vi "Z_valve_state.vi"(0 "Z_Source":T1(ring), 1 "ZM_State":u32, 5 "Z_SetState":T2(ring)=enum."on", 7 "Alarm_L1":bool, 9 "Alarm_L2":bool, 12 "TsStop":u32=1000, 13 "t_check":u32=10000) -> (4 "Z_Source_Out":T1(ring), 6 "Z_State":T2(ring), 8 "t":u32)   [LabVIEW 2019, in "Valves.lvlib"]
uses:
  Valves.lvlib
  Trigers/RS.vi
  Timer Delay/Timer.vi
  Userlib.lvlib
panel:
  in  "t2_tmp":u32[][](array[numeric])=[[0, 0], [0, 0], [0, 0], [0, 0], [0, 0], [0, 0], [0, 0], [0, 0], [0, 0], [0, 0], [0, 0], [0, 0], [0, 0]]
  in  "C2_tmp":cluster{"C":bool, "NC":u32}[][](array[cluster])
  in  "t_tmp":u32[][](array[numeric])=[[0, 0], [0, 0], [0, 0], [0, 0], [0, 0], [0, 0], [0, 0], [0, 0], [0, 0], [0, 0], [0, 0], [0, 0], [0, 0]]
  in  "C_tmp":cluster{"C":bool, "NC":u32}[][](array[cluster])
  # "Temporally arrays"
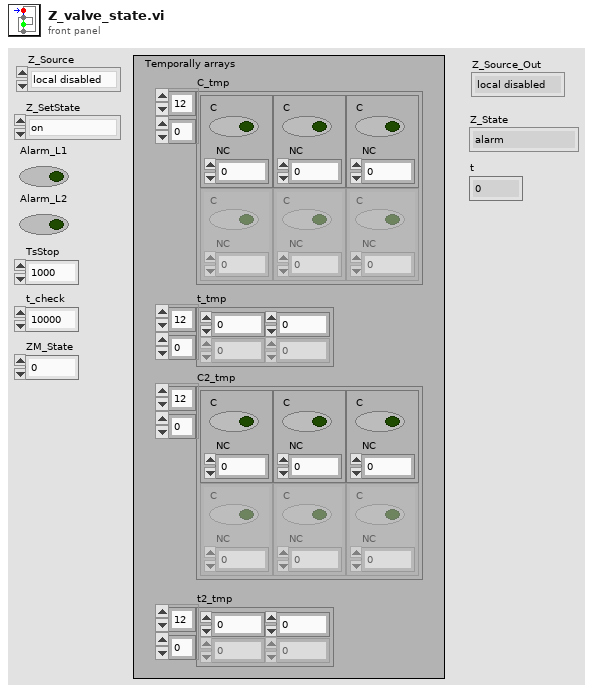
[diagram p1: front panel]
types:
  T1 = enum8{"local disabled", "local hand", "hand", "auto", "dist"}
  T2 = enum8{"alarm", "disabled", "not ready", "stop ready", "reserv", "switched off", "switched on", "check", "on min", "decrease speed", "on", "increase speed", "on max"}
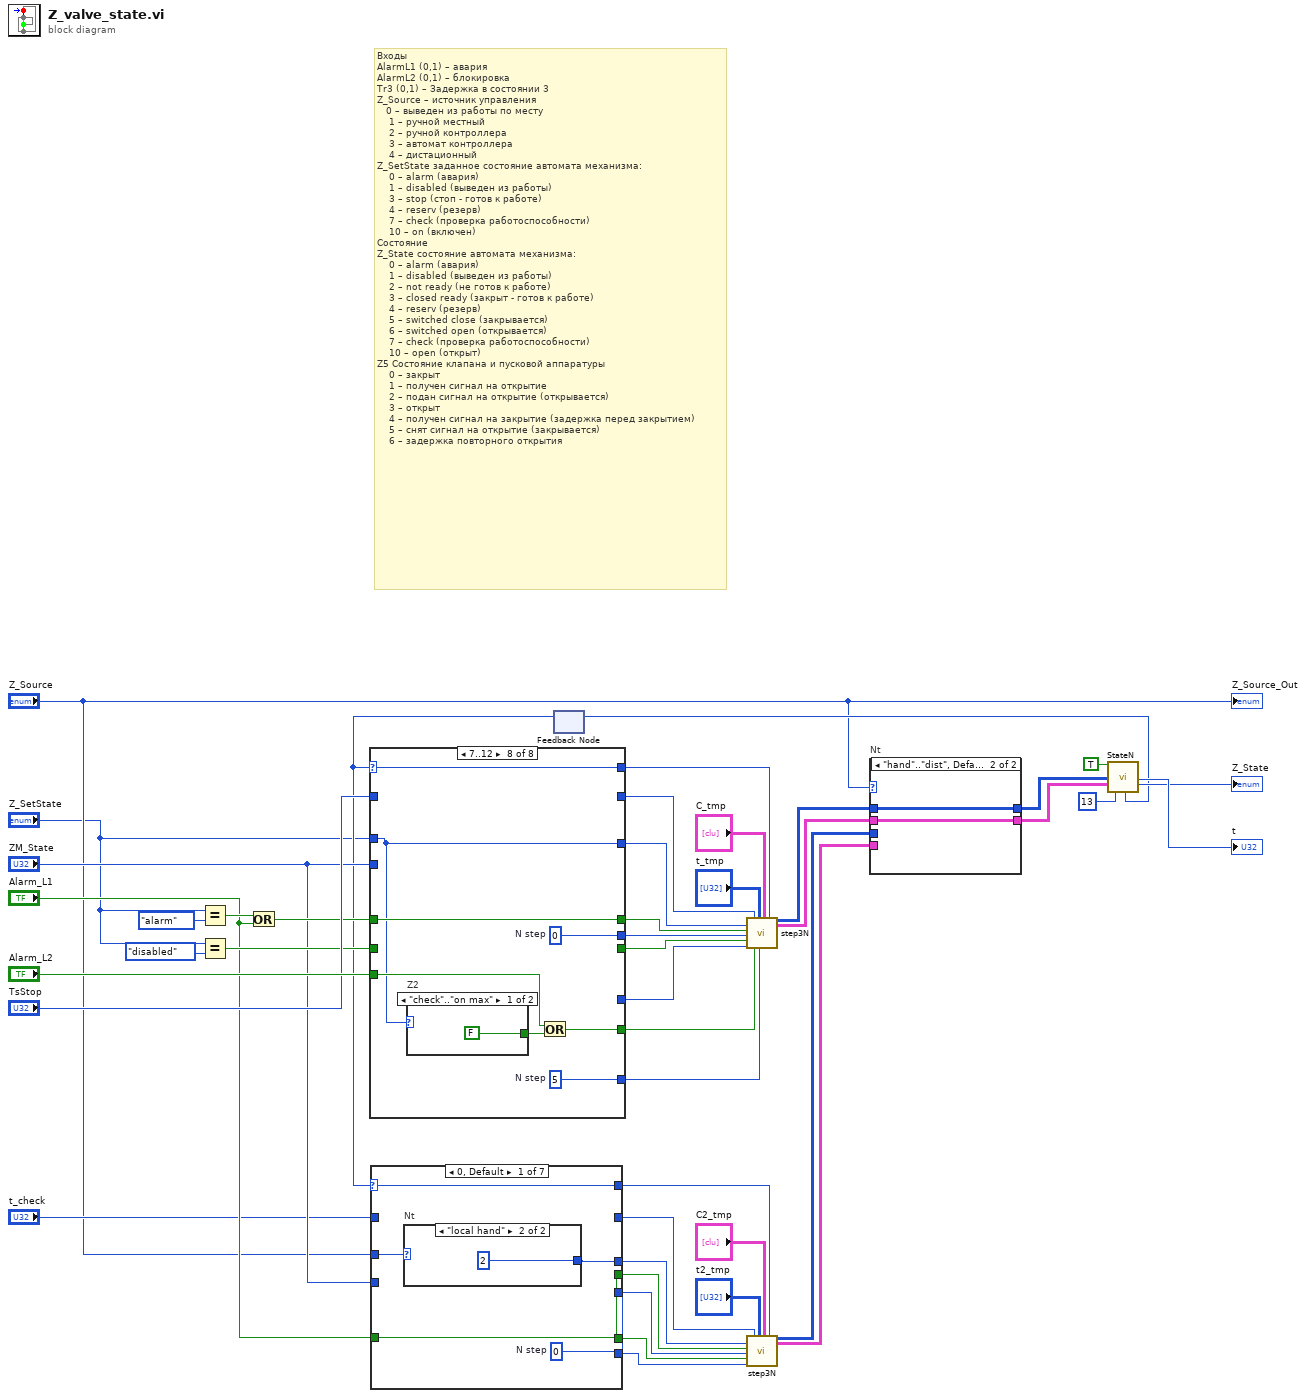
[diagram p0: block diagram]
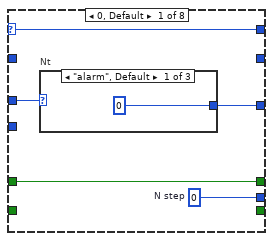
[diagram p2: hidden frame]
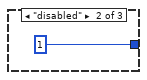
[diagram p3: hidden frame]
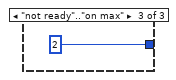
[diagram p4: hidden frame]
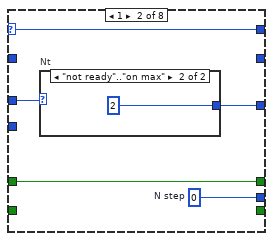
[diagram p5: hidden frame]
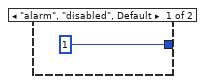
[diagram p6: hidden frame]
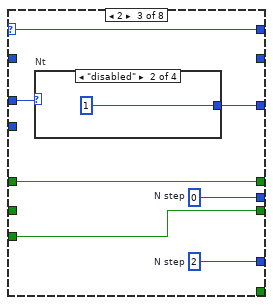
[diagram p7: hidden frame]
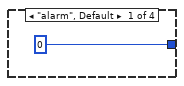
[diagram p8: hidden frame]
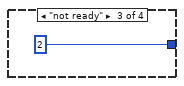
[diagram p9: hidden frame]
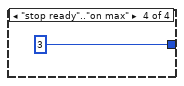
[diagram p10: hidden frame]
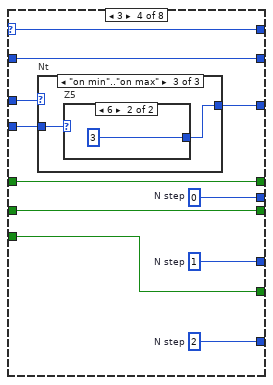
[diagram p11: hidden frame]
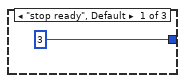
[diagram p12: hidden frame]
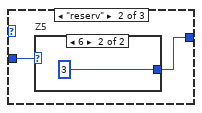
[diagram p13: hidden frame]
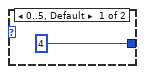
[diagram p14: hidden frame]
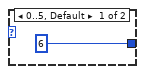
[diagram p15: hidden frame]
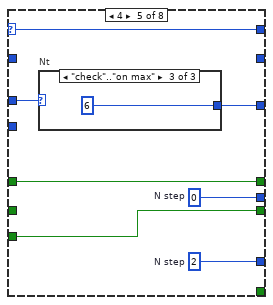
[diagram p16: hidden frame]
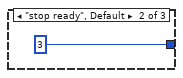
[diagram p18: hidden frame]
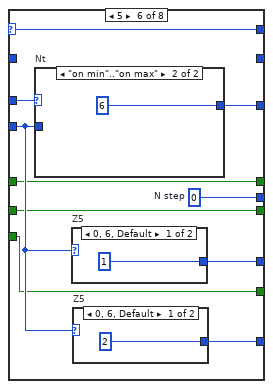
[diagram p19: hidden frame]
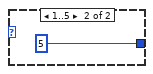
[diagram p20: hidden frame]
diagram:
  # "Входы\nAlarmL1 (0,1) – авария\nAlarmL2 (0,1) – блокировка\nTr3 (0,1) – Задержка в состоянии 3\nZ_Source – источник управления\n   0 – выведен из работы по месту\n    1 – ручной местный\n    2 – ручной контроллера\n    3 – автомат контроллера\n    4 – дистационный\nZ_SetState заданное состояние автомата механизма:\n    0 – alarm (авария)\n    1 – disabled (выведен из работы)\n    3 – stop (стоп - готов к работе)\n    4 – reserv (резерв)\n    7 – check (проверка работоспособности)\n    10 – on (включен)\nСостояние\nZ_State состояние автомата механизма:\n    0 – alarm (авария)\n    1 – disabled (выведен из работы)\n    2 – not ready (не готов к работе)\n    3 – closed ready (закрыт - готов к работе)\n    4 – reserv (резерв)\n    5 – switched close (закрывается)\n    6 – switched open (открывается)\n    7 – check (проверка работоспособности)\n    10 – open (открыт)\nZ5 Состояние клапана и пусковой аппаратуры\n    0 – закрыт\n    1 – получен сигнал на открытие\n    2 – подан сигнал на открытие (открывается)\n    3 – открыт\n    4 – получен сигнал на закрытие (задержка перед закрытием)\n    5 – снят сигнал на открытие (закрывается)\n    6 – задержка повторного открытия"
  n1 = Equal?(x="Z_SetState", y=T2."alarm") -> (x = y?=w44:bool)
  n2 = Equal?(x="Z_SetState", y=T2."disabled") -> (x = y?=w33:bool)
  n3 = Or(x=w44, y="Alarm_L1") -> (x .or. y?=w32:bool)
  n4 = feedback #1() -> (w7:u32)  [unwired: 1 in]
  n5 = case shown="7..12" w7 {
    selector: w7 -> [w47 w55 w62 w80 w97 w102 w126 w135]
    tunnel: w32 -> [w48 w56 w63 w73 w92 w103 w121 w139]
    tunnel: "Alarm_L2" -> [_ _ w65 w77 w94 w107 w127 w141]
    tunnel: "ZM_State" -> [_ _ _ w81 _ w110 w129 _]
    tunnel: "TsStop" -> [_ _ _ w79 _ _ _ _]
    tunnel: w33 -> [_ _ _ w75 _ w105 _ _]
    tunnel: [w47 w55 w62 w80 w97 w102 w126 w135] -> w18
    tunnel: [w48 w56 w63 w73 w92 w103 w121 w139] -> w25
    tunnel: [w49 w57 w64 w74 w93 w104 w122 w138] -> w24
    tunnel: [_ _ _ w77 _ w107 w124 w137] -> w20
    tunnel: [_ _ _ w78 _ w108 w123 w136] -> w19
    tunnel: [w46 w54 w61 w72 w96 w109 w125 w134] -> w23
    tunnel: [_ _ w66 w76 w95 w106 _ _] -> w22
    tunnel: [_ _ w65 w75 w94 w105 _ _] -> w21
    tunnel: [_ _ _ w79 _ _ _ _] -> w17
    tunnel: "Z_SetState" -> [w45 w53 w60 w71 w91 w101 w120 w134]
    frame 0, Default {
      w49 = u32 0  # N step
      n6 = case "Nt" shown="\"alarm\", Default" w45 {
        tunnel: [u32 0 ("End step") u32 1 ("End step") u32 2 ("End step")] -> w46
        frame "alarm", Default {
        }
        frame "disabled" {
        }
        frame "not ready".."on max" {
        }
      }
    }
    frame 1 {
      w57 = u32 0  # N step
      n7 = case "Nt" shown="\"not ready\"..\"on max\"" w53 {
        tunnel: [u32 1 ("End step") u32 2 ("End step")] -> w54
        frame "alarm", "disabled", Default {
        }
        frame "not ready".."on max" {
        }
      }
    }
    frame 2 {
      w66 = u32 2  # N step
      w64 = u32 0  # N step
      n8 = case "Nt" shown="\"disabled\"" w60 {
        tunnel: [u32 0 ("End step") u32 1 ("End step") u32 2 ("End step") u32 3 ("End step")] -> w61
        frame "alarm", Default {
        }
        frame "disabled" {
        }
        frame "not ready" {
        }
        frame "stop ready".."on max" {
        }
      }
    }
    frame 3 {
      w78 = u32 2  # N step
      w76 = u32 1  # N step
      w74 = u32 0  # N step
      n9 = case "Nt" shown="\"on min\"..\"on max\"" w71 {
        tunnel: [u32 3 ("End step") w83 w87] -> w72
        tunnel: w81 -> [_ w84 w88]
        frame "stop ready", Default {
        }
        frame "reserv" {
          n10 = case "Z5" shown="6" w84 {
            tunnel: [u32 4 ("End step") u32 3 ("End step")] -> w83
            frame 0..5, Default {
            }
            frame 6 {
            }
          }
        }
        frame "on min".."on max" {
          n11 = case "Z5" shown="6" w88 {
            tunnel: [u32 6 ("End step") u32 3 ("End step")] -> w87
            frame 0..5, Default {
            }
            frame 6 {
            }
          }
        }
      }
    }
    frame 4 {
      w95 = u32 2  # N step
      w93 = u32 0  # N step
      n12 = case "Nt" shown="\"check\"..\"on max\"" w91 {
        selector: w91 -> [w98 _ _]
        tunnel: [w98 u32 3 ("End step") u32 6 ("End step")] -> w96
        frame "alarm".."not ready", "reserv" {
        }
        frame "stop ready", Default {
        }
        frame "check".."on max" {
        }
      }
    }
    frame 5 {
      w104 = u32 0  # N step
      n13 = case "Nt" shown="\"on min\"..\"on max\"" w101 {
        tunnel: [w115 u32 6 ("End step")] -> w109
        tunnel: w110 -> [w116 _]
        frame "stop ready", "reserv", "check", Default {
          n14 = case "Z5" shown="1..5" w116 {
            tunnel: [u32 3 ("End step") u32 5 ("End step")] -> w115
            frame 0, 6, Default {
            }
            frame 1..5 {
            }
          }
        }
        frame "on min".."on max" {
        }
      }
      n15 = case "Z5" shown="0, 6, Default" w110 {
        tunnel: [u32 1 ("End step") u32 5 ("End step")] -> w106
        frame 0, 6, Default {
        }
        frame 1..5 {
        }
      }
      n16 = case "Z5" shown="0, 6, Default" w110 {
        tunnel: [u32 2 ("End step") u32 5 ("End step")] -> w108
        frame 0, 6, Default {
        }
        frame 1..5 {
        }
      }
    }
    frame 6 {
      w123 = u32 5  # N step
      w122 = u32 0  # N step
      n17 = case "Z5" shown="3" w129 {
        tunnel: [u32 6 ("End step") w133] -> w125
        tunnel: w120 -> [_ w133]
        frame 0..2, Default {
        }
        frame 3 {
        }
      }
      n18 = case "Z2" shown="\"check\"..\"on max\"" w120 {
        tunnel: [FALSE TRUE] -> w128
        frame "check".."on max" {
        }
        frame "disabled".."reserv", Default {
        }
      }
      n19 = Or(x=w127, y=w128) -> (x .or. y?=w124:bool)
    }
    frame 7..12 {
      w136 = u32 5  # N step
      w138 = u32 0  # N step
      n20 = case "Z2" shown="\"check\"..\"on max\"" w134 {
        tunnel: [FALSE TRUE] -> w140
        frame "check".."on max" {
        }
        frame "disabled".."reserv", Default {
        }
      }
      n21 = Or(x=w141, y=w140) -> (x .or. y?=w137:bool)
    }
  }
  n22 = case shown="0, Default" w7 {
    selector: w7 -> [w147 w152 w159 w170 w182 w193 w205]
    tunnel: "Alarm_L1" -> [w145 _ w156 w168 w180 w190 w202]
    tunnel: "ZM_State" -> [_ _ w160 w171 w183 w194 w206]
    tunnel: "Z_Source" -> [w148 w153 w161 w172 _ _ _]
    tunnel: "t_check" -> [_ _ _ _ _ w192 w204]
    tunnel: [w147 w152 w159 w170 w182 w193 w205] -> w16
    tunnel: [_ _ _ _ _ w192 w204] -> w13
    tunnel: [_ _ _ _ _ w191 _] -> w12
    tunnel: [_ _ _ _ _ w190 _] -> w11
    tunnel: [w144 _ w157 w167 w179 w188 w201] -> w10
    tunnel: [w145 _ w156 w168 w180 w189 w202] -> w9
    tunnel: [w146 w151 w158 w169 w181 w188 w203] -> w8
    frame 0, Default {
      w144 = u32 0  # N step
      n23 = case "Nt" shown="\"local hand\"" w148 {
        tunnel: [u32 1 ("End step") u32 2 ("End step")] -> w146
        frame "local disabled", Default {
        }
        frame "local hand" {
        }
      }
    }
    frame 1, 3, 4 {
      n24 = case "Nt" shown="\"local hand\"" w153 {
        tunnel: [u32 1 ("End step") u32 2 ("End step")] -> w151
        frame "local disabled", Default {
        }
        frame "local hand" {
        }
      }
    }
    frame 2 {
      w157 = u32 0  # N step
      n25 = case "Nt" shown="\"local disabled\", Default" w161 {
        tunnel: [u32 1 ("End step") w164] -> w158
        tunnel: w160 -> [_ w163]
        frame "local disabled", Default {
        }
        frame "local hand" {
          n26 = case "Z5" shown="0, 1, 4..6, Default" w163 {
            tunnel: [u32 2 ("End step") u32 6 ("End step")] -> w164
            frame 0, 1, 4..6, Default {
            }
            frame 2, 3 {
            }
          }
        }
      }
    }
    frame 5 {
      w167 = u32 0  # N step
      n27 = case "Nt" shown="\"local hand\", Default" w172 {
        tunnel: [u32 1 ("End step") w174] -> w169
        tunnel: w171 -> [_ w175]
        frame "local disabled" {
        }
        frame "local hand", Default {
          n28 = case "Z5" shown="0, 6, Default" w175 {
            tunnel: [u32 2 ("End step") u32 6 ("End step") u32 5 ("End step")] -> w174
            frame 0, 6, Default {
            }
            frame 2, 3 {
            }
            frame 1, 4, 5 {
            }
          }
        }
      }
    }
    frame 6 {
      w179 = u32 0  # N step
      n29 = case "Z5" shown="0, 6, Default" w183 {
        tunnel: [u32 2 ("End step") u32 6 ("End step") u32 7 ("End step") u32 5 ("End step")] -> w181
        frame 0, 6, Default {
        }
        frame 1, 2 {
        }
        frame 3 {
        }
        frame 4, 5 {
        }
      }
    }
    frame 7 {
      w191 = u32 0  # N step
      n30 = case "Z5" shown="0, Default" w194 {
        tunnel: [u32 2 ("End step") u32 10 ("End step") u32 5 ("End step")] -> w188
        tunnel: [TRUE FALSE TRUE] -> w189
        frame 0, Default {
        }
        frame 1..4 {
        }
        frame 5, 6 {
        }
      }
    }
    frame 8..12 {
      w201 = u32 0  # N step
      n31 = case "Z5" shown="0, Default" w206 {
        tunnel: [u32 2 ("End step") u32 10 ("End step") u32 5 ("End step")] -> w203
        frame 0, Default {
        }
        frame 1..4 {
        }
        frame 5, 6 {
        }
      }
    }
  }
  n32 = call "step3N.vi"("NT"=w23, "C1"=w25, "NC1"=w24, "C2"=w21, "NC2"=w22, "T"=w17, "C3"=w20, "T NT2"="t_tmp", "NC3"=w19, "C NC2"="C_tmp", "N step"=w18) -> ("T NT"=w28:u32[][], "C NC"=w27:cluster{"C":bool, "NC":u32}[][])  [unwired: 7 in]
  n33 = call "step3N.vi"("NT"=w8, "C1"=w9, "NC1"=w10, "C2"=w11, "NC2"=w12, "T"=w13, "T NT2"="t2_tmp", "C NC2"="C2_tmp", "N step"=w16) -> ("T NT"=w15:u32[][], "C NC"=w14:cluster{"C":bool, "NC":u32}[][])  [unwired: 9 in]
  n34 = case "Nt" shown="\"hand\"..\"dist\", Default" "Z_Source" {
    tunnel: w28 -> [_ w213]
    tunnel: w27 -> [_ w212]
    tunnel: [w211 w213] -> w40
    tunnel: [w210 w212] -> w39
    tunnel: w15 -> [w211 _]
    tunnel: w14 -> [w210 _]
    frame "local disabled", "local hand" {
    }
    frame "hand".."dist", Default {
    }
  }
  n35 = call "StateN.vi"("Start"=TRUE, "T_table"=w40, "C_table"=w39, "End step"=u32 13) -> ("N next"=w26:u32, "t"=→"t":u32, "N curr"=→"Z_State":u32)  [unwired: 10 in, 3 out]
  n36 = feedback-in #1(w26) -> ()
  "Z_Source_Out" <- "Z_Source"
